vi "GRIPPER.vi"() -> ()   [LabVIEW 2016]
uses:
  <vilib>/myRIO/Instrument Drivers/Onboard IO/DIO/typedefs/DIO Reference.ctl
  <vilib>/myRIO/Common/Instrument Driver Framework/Utilities/typedefs/myRIO Generic Hardware Reference.ctl
  <vilib>/myRIO/Common/Instrument Driver Framework/Utilities/typedefs/Hardware Version Enum.ctl
  <vilib>/myRIO/Common/Instrument Driver Framework/Utilities/typedefs/myRIO v1.0 Reference.ctl
  <vilib>/myRIO/Common/Instrument Driver Framework/Utilities/typedefs/Generic FPGA Reference.ctl
  <vilib>/myRIO/Common/Instrument Driver Framework/myRIO v1.0/DIO/typedefs/DIO Channels List.ctl
  <vilib>/myRIO/Common/Instrument Driver Framework/myRIO v1.0/DIO/typedefs/DIO Channels Enum.ctl
  <vilib>/userdefined/High Color/nirio_resource_hc.ctl
  <vilib>/myRIO/Instrument Drivers/Onboard IO/AI/typedefs/AI Reference.ctl
  <vilib>/myRIO/Common/Instrument Driver Framework/myRIO v1.0/AI/typedefs/AI Channels List.ctl
  <vilib>/myRIO/Common/Instrument Driver Framework/myRIO v1.0/AI/typedefs/AI Channels Enum.ctl
  <vilib>/myRIO/Common/Instrument Driver Framework/Utilities/typedefs/Analog Scaling Constants List.ctl
  <vilib>/myRIO/Common/Instrument Driver Framework/Utilities/typedefs/Analog Scaling Constants.ctl
  <vilib>/myRIO/Common/Instrument Driver Framework/Utilities/vis/Is FPGA Ref Available.vi
  <vilib>/myRIO/Common/Instrument Driver Framework/myRIO v1.0/AI/vis/myRIO v1.1 Open AI.vi
  <vilib>/myRIO/Instrument Drivers/Onboard IO/AI/vis/Read.vi
  <vilib>/myRIO/Common/Instrument Driver Framework/myRIO v1.0/DIO/vis/myRIO v1.1 Open DIO.vi
  <vilib>/myRIO/Instrument Drivers/Onboard IO/DIO/vis/Write.vi
  <vilib>/myRIO/Common/Instrument Driver Framework/Utilities/vis/Validate Channels.vi
  <vilib>/myRIO/Common/Instrument Driver Framework/myRIO v1.0/AI/vis/myRIO v1.0 Reserve AI.vi
  <vilib>/myRIO/Common/Instrument Driver Framework/myRIO v1.0/DIO/vis/myRIO v1.0 Reserve DIO.vi
  <vilib>/myRIO/Common/Instrument Driver Framework/myRIO v1.0/PWM/vis/myRIO v1.1 Open PWM.vi
  <vilib>/myRIO/Common/Instrument Driver Framework/myRIO v1.0/UART/vis/myRIO v1.0 Close UART.vi
  <vilib>/myRIO/Common/Instrument Driver Framework/myRIO v1.0/AI/vis/myRIO v1.0 Build MUX Configuration AI.vi
  <vilib>/myRIO/Common/Instrument Driver Framework/myRIO v1.0/Resource Manager/vis/myRIO v1.0 Reserve Channel List.vi
  <vilib>/myRIO/Common/Instrument Driver Framework/myRIO v1.0/DIO/vis/myRIO v1.0 Build MUX Configuration DIO.vi
  <vilib>/myRIO/Common/Instrument Driver Framework/myRIO v1.0/PWM/vis/myRIO v1.0 Reserve PWM.vi
  <vilib>/myRIO/Common/Instrument Driver Framework/myRIO v1.0/Resource Manager/vis/myRIO v1.0 Reserve Channel.vi
  <vilib>/myRIO/Common/Instrument Driver Framework/myRIO v1.0/Resource Manager/vis/myRIO v1.0 Unreserve Channel.vi
  <vilib>/myRIO/Common/Instrument Driver Framework/myRIO v1.0/Resource Manager/vis/myRIO v1.0 Create Configuration List.vi
  <vilib>/myRIO/Common/Instrument Driver Framework/myRIO v1.0/PWM/vis/myRIO v1.0 Build MUX Configuration PWM.vi
  <vilib>/myRIO/Common/Instrument Driver Framework/myRIO v1.0/Resource Manager/vis/myRIO v1.0 Build Mutex Name.vi
  <vilib>/Utility/VariantDataType/GetNumericInfo.vi
  <vilib>/Utility/error.llb/Error Cluster From Error Code.vi
  <vilib>/myRIO/Common/Instrument Driver Framework/myRIO v1.0/myRIO v1.1 Open.vi
  <vilib>/myRIO/Common/Instrument Driver Framework/Utilities/vis/IO Manager.vi
  <vilib>/myRIO/Common/Instrument Driver Framework/Utilities/vis/Configuration Manager.vi
  <vilib>/myRIO/Common/Instrument Driver Framework/myRIO v1.0/Resource Manager/vis/myRIO v1.0 Configure IO.vi
  <vilib>/myRIO/Common/Instrument Driver Framework/myRIO v1.0/myRIO v1.0 Close.vi
  <vilib>/myRIO/Common/Instrument Driver Framework/myRIO v1.0/DIO/vis/myRIO v1.0 Write DIO.vi
  <vilib>/myRIO/Common/Instrument Driver Framework/myRIO v1.0/PWM/vis/myRIO v1.0 Write PWM.vi
  <vilib>/myRIO/Common/Instrument Driver Framework/myRIO v1.0/AI/vis/myRIO v1.0 Get Scaling Constants AI.vi
  <vilib>/myRIO/Common/Instrument Driver Framework/myRIO v1.0/AI/vis/myRIO v1.0 Read AI.vi
  <vilib>/myRIO/Common/Instrument Driver Framework/Utilities/vis/FPGA Ref Manager.vi
  <vilib>/myRIO/Common/Instrument Driver Framework/myRIO v1.0/myRIO v1.0 Reset FPGA.vi
  <vilib>/myRIO/Common/Instrument Driver Framework/myRIO v1.0/IRQ/vis/myRIO v1.0 IRQ Info FGV.vi
  <vilib>/myRIO/Common/Instrument Driver Framework/myRIO v1.0/IRQ/vis/myRIO v1.0 Timer IRQ Info FGV.vi
  <vilib>/myRIO/Common/Instrument Driver Framework/myRIO v1.0/IRQ/vis/myRIO v1.0 ISR Agent.vi
  <vilib>/myRIO/Express VI/Onboard IO/DO/DO Express VI.xnode
  <vilib>/myRIO/Instrument Drivers/Onboard IO/DIO/vis/myRIO DIO Open.xnode
  <vilib>/myRIO/Express VI/Onboard IO/AI/AI Express VI.xnode
  <vilib>/myRIO/Instrument Drivers/Onboard IO/AI/vis/myRIO AI Open.xnode
  <vilib>/myRIO/Instrument Drivers/Onboard IO/DIO/DIO.lvlib
  <vilib>/myRIO/Instrument Drivers/Onboard IO/AI/AI.lvlib
  <vilib>/myRIO/Instrument Drivers/Onboard IO/PWM/PWM.lvlib
  <vilib>/myRIO/Instrument Drivers/Utilities/Utilities.lvlib
panel:
  out "FSR 2":bool
  in  "Boolean":bool
  in  "milliseconds to wait 5":u32
  out "left fsr (A/AI1 (Pin 5))":dbl
  in  "Servo":bool
  in  "PWM channel":tag="B/PWM0"
  out "position [%FS]":dbl(slide) scale=0.0..180.0 scale format="%#_5g"
  out "pulse width [ms]":dbl=1.5
  out "duty cycle [%]":dbl
  in  "Stop Button":bool
  out "B/AI0 (Pin 3)":dbl
  out "Knob":dbl(knob) scale=0.0..4.0
  out "C Count":dbl
  out "A":bool
  out "C 2":bool
  out "D":bool
  out "B":bool
  in  "DIRECTION":bool
  in  "DRIVE":bool
  out "CC Count":dbl
  # "WHEN  THE DIRECTION BUTTON IS PRESSED \nTHE ROTATION IS COUNTER-CLOCK WISE"
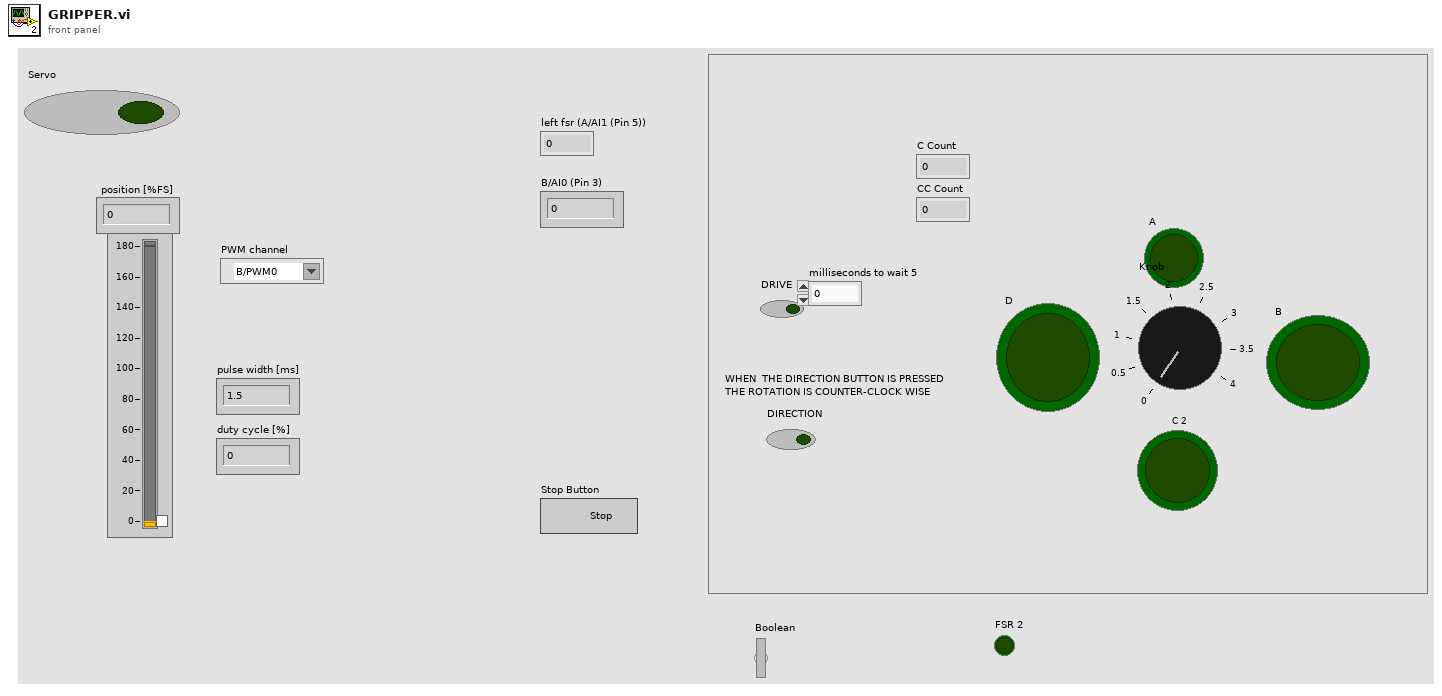
[diagram p1: front panel]
types:
  T1 = typedef "DIO.lvlib/DIO Reference.ctl" = cluster{"myRIO Reference":T2, "DIO Channels List":T6}
  T2 = typedef "myRIO Generic Hardware Reference.ctl" = cluster{"myRIO Model":T3, "myRIO Hardware Reference":T4}
  T3 = typedef "Hardware Version Enum.ctl" = enum16{"Unknown", "myRIO-1900", "myRIO-1950", "roboRIO", "NI ELVIS RIO CM"}
  T4 = typedef "myRIO v1.0 Reference.ctl" = cluster{"Generic FPGA Reference":T5, "Allow multiple opens":bool}
  T5 = typedef "Generic FPGA Reference.ctl" = refnum<k20>
  T6 = typedef "DIO Channels List.ctl" = T7[]
  T7 = typedef "DIO Channels Enum.ctl" = enum16{"Not Connected", "C/DIO0", "C/DIO1", "C/DIO2", "C/DIO3", "C/DIO4", "C/DIO5", "C/DIO6", "C/DIO7", "A/DIO0", "A/DIO1", "A/DIO2", "A/DIO3", "A/DIO4", "A/DIO5", "A/DIO6", "A/DIO7", "A/DIO8", "A/DIO9", "A/DIO10", "A/DIO11", "A/DIO12", "A/DIO13", "A/DIO14", "A/DIO15", "B/DIO0", "B/DIO1", "B/DIO2", "B/DIO3", "B/DIO4", "B/DIO5", "B/DIO6", "B/DIO7", "B/DIO8", "B/DIO9", "B/DIO10", "B/DIO11", "B/DIO12", "B/DIO13", "B/DIO14", "B/DIO15", "LED0", "LED1", "LED2", "LED3", "Button0", "DIO/DIO0", "DIO/DIO1", "DIO/DIO2", "DIO/DIO3", "DIO/DIO4", "DIO/DIO5", "DIO/DIO6", "DIO/DIO7", "DIO/DIO8", "DIO/DIO9", "SPI/CS0", "SPI/CS1", "SPI/CS2", "SPI/CS3", "LED RADIO (Green)", "LED RADIO (Red)", "LED COMM (Green)", "LED COMM (Red)", "LED MODE (Green)", "LED MODE (Red)"}
  T8 = typedef "nirio_resource_hc.ctl" = tag
  T9 = typedef "AI.lvlib/AI Reference.ctl" = cluster{"myRIO Reference":T2, "AI Channels List":T10, "AI Scaling Constants List":T12}
  T10 = typedef "AI Channels List.ctl" = T11[]
  T11 = typedef "AI Channels Enum.ctl" = enum16{"Not Connected", "AudioIn/Left", "AudioIn/Right", "C/AI0", "C/AI1", "A/AI0", "A/AI1", "A/AI2", "A/AI3", "B/AI0", "B/AI1", "B/AI2", "B/AI3", "AI/AI0", "AI/AI1", "AI/AI2", "AI/AI3"}
  T12 = typedef "Analog Scaling Constants List.ctl" = T13[]
  T13 = typedef "Analog Scaling Constants.ctl" = cluster{"LSB Weight (Volts)":dbl, "Offset (Volts)":dbl, "Signed?":bool}
  T14 = typedef "PWM.lvlib/PWM Reference.ctl" = cluster{"myRIO Reference":T2, "PWM Channels Enum":T15, "PWM Configuration":T16}
  T15 = typedef "PWM Channels Enum.ctl" = enum16{"Not Connected", "C/PWM0", "C/PWM1", "A/PWM0", "A/PWM1", "A/PWM2", "B/PWM0", "B/PWM1", "B/PWM2", "PWM/PWM0", "PWM/PWM1", "PWM/PWM2", "PWM/PWM3", "PWM/PWM4", "PWM/PWM5", "PWM/PWM6", "PWM/PWM7", "PWM/PWM8", "PWM/PWM9"}
  T16 = typedef "PWM.lvlib/PWM Configuration.ctl" = cluster{"Frequency":dbl, "Duty Cycle":dbl}
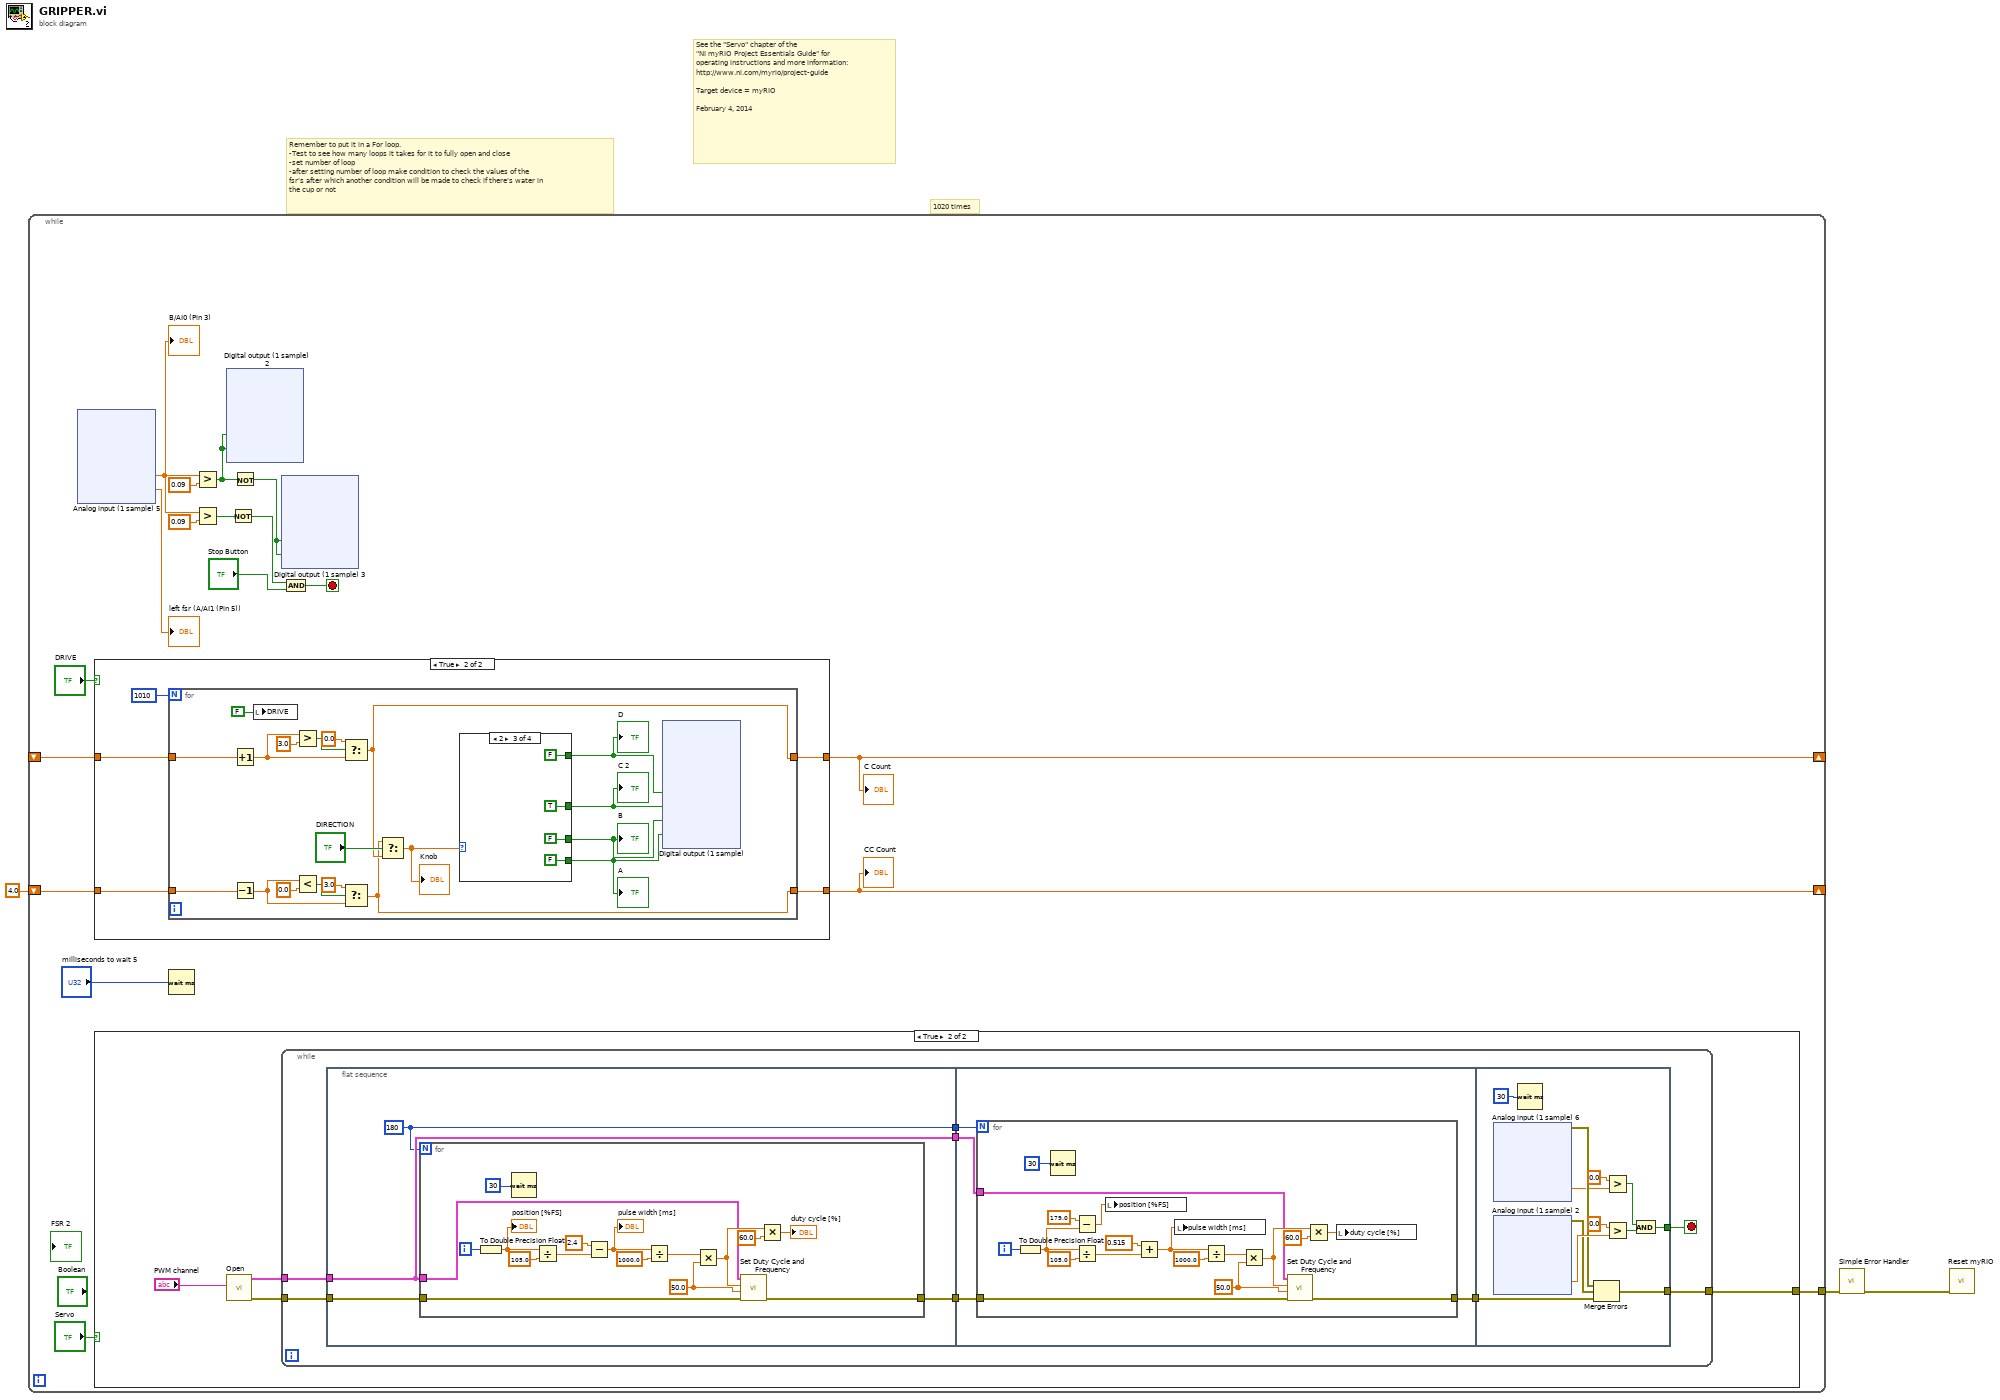
[diagram p0: block diagram]
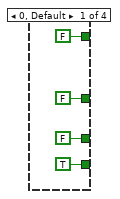
[diagram p3: hidden frame]
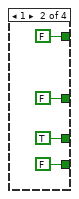
[diagram p4: hidden frame]
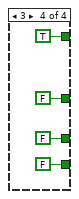
[diagram p5: hidden frame]
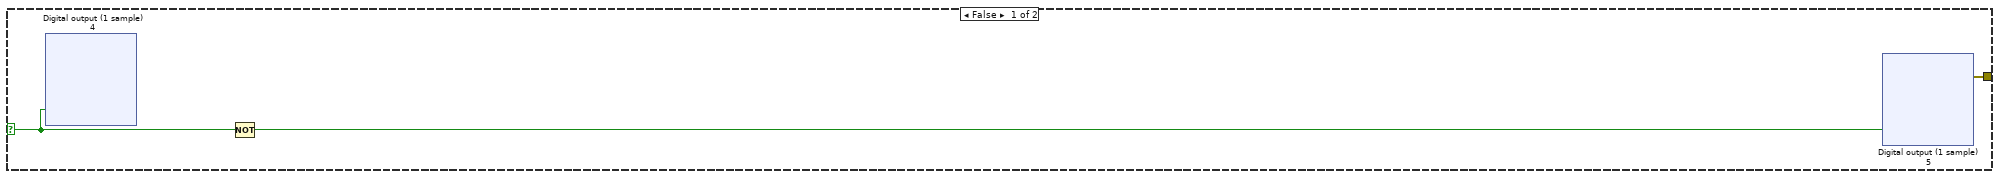
[diagram p6: hidden frame]
diagram:
  # "1020 times"
  # "Remember to put it in a For loop.\n-Test to see how many loops it takes for it to fully open and close\n-set number of loop\n-after setting number of loop make condition to check the values of the \nfsr's after which another condition will be made to check if there's water in \nthe cup or not"
  # "See the \"Servo\" chapter of the\n\"NI myRIO Project Essentials Guide\" for\noperating instructions and more information: \nhttp://www.ni.com/myrio/project-guide\n\nTarget device = myRIO\n\nFebruary 4, 2014"
  n1 = while {
    tunnel: [w21] -> w2
    shift-right: [w7] -> _
    shift-left: 4.0 -> [w20]
    shift-right: [w4] -> _
    shift-left: _ -> [w19]
    stop <- w13 stop-if-true
    n2 = xnode "Analog input (1 sample) 5"() -> ("right fsr (A/AI0 (Pin 3))"=w9:dbl, "left fsr (A/AI1 (Pin 5))"=→"left fsr (A/AI1 (Pin 5))":dbl)  [unwired: 1 in, 1 out]
    "B/AI0 (Pin 3)" <- w9
    n3 = case shown="True" "DRIVE" {
      tunnel: w20 -> [w23 w28]
      tunnel: w19 -> [w22 w27]
      tunnel: [w22 w26] -> w4
      tunnel: [w23 w25] -> w7
      frame False {
      }
      frame True {
        n4 = for {
          N: 1010 -> [_]
          tunnel: w28 -> [w33]
          tunnel: w27 -> [w32]
          tunnel: [w31] -> w26
          tunnel: [w30] -> w25
          n5 = Increment(x=w32) -> (x+1=w39:dbl)
          n6 = Decrement(x=w33) -> (x-1=w40:dbl)
          n7 = local write "DRIVE"(FALSE) -> ()
          n8 = Greater?(x=w39, y=3.0) -> (0:w43:bool)
          n9 = Less?(x=w40, y=0.0) -> (x < y?=w46:bool)
          n10 = Select(t=0.0, s=w43, f=w39) -> (s? t:f=w31:dbl)
          n11 = Select(t=3.0, s=w46, f=w40) -> (s? t:f=w30:dbl)
          n12 = Select(t=w30, s="DIRECTION", f=w31) -> (s? t:f=w34:dbl)
          "Knob" <- w34
          n13 = case shown="2" w34 {
            tunnel: [TRUE FALSE FALSE FALSE] -> w38
            tunnel: [FALSE FALSE FALSE TRUE] -> w35
            tunnel: [FALSE FALSE TRUE FALSE] -> w36
            tunnel: [FALSE TRUE FALSE FALSE] -> w37
            frame 0, Default {
            }
            frame 1 {
            }
            frame 2 {
            }
            frame 3 {
            }
          }
          "A" <- w38
          "C 2" <- w36
          "D" <- w35
          "B" <- w37
          n14 = xnode "Digital output (1 sample)"("IN4 (A/DIO10 (Pin 31))"=w35, "IN3 (A/DIO11 (Pin 18))"=w36, "IN2 (A/DIO13 (Pin 26))"=w37, "IN1 (A/DIO15 (Pin 34))"=w38) -> ()  [unwired: 1 in, 1 out]
        }
      }
    }
    "C Count" <- w4
    "CC Count" <- w7
    n15 = case shown="True" "Servo" {
      selector: "Servo" -> [w212 _]
      tunnel: [w213 w286] -> w21
      frame False {
        n16 = xnode "Digital output (1 sample) 4"("B/DIO15 (Pin 34)"=w212) -> ()  [unwired: 1 in, 1 out]
        n17 = Not(x=w212) -> (.not. x?=w214:bool)
        n18 = xnode "Digital output (1 sample) 5"("B/DIO14 (Pin 32)"=w214) -> ("error out"=w213:errorcluster)  [unwired: 1 in]
      }
      frame True {
        n19 = call <vilib>:"Open.vi"("Channel Name"="PWM channel") -> ("error out"=w285:errorcluster, "PWM Ref Out"=w287:T14)  [unwired: 9 in]
        n20 = while {
          tunnel: w287 -> [w296]
          tunnel: [w291] -> w286
          tunnel: w285 -> [w295]
          stop <- w289 stop-if-true
          n21 = flat-sequence {
            tunnel: w296 -> [w298]
            tunnel: w295 -> [w299]
            tunnel: [w300] -> w294
            tunnel: [w298] -> w293
            tunnel: [w297] -> w292
            tunnel: w294 -> [w318]
            tunnel: w293 -> [w320]
            tunnel: w292 -> [w319]
            tunnel: [w317] -> w290
            tunnel: [w344] -> w291
            tunnel: w290 -> [w345]
            tunnel: [w348] -> w289
            frame #0 {
              w297 = 180
              n22 = for {
                N: w297 -> [_]
                tunnel: [w312] -> w300
                tunnel: w298 -> [w304]
                tunnel: w299 -> [w301]
                i -> [w302]
                w313 = 50.0 ("freq [Hz]")
                n23 = To Double Precision Float(number=w302) -> (double precision float=w305:dbl)
                "position [%FS]" <- w305
                n24 = Wait (ms)(milliseconds to wait=u32 30) -> ()  [unwired: 1 out]
                n25 = Divide(x=w305, y=105.0) -> (x/y=w307:dbl)
                n26 = Subtract(x=2.4 ("y"), y=w307) -> (x-y=w303:dbl)
                "pulse width [ms]" <- w303
                n27 = Divide(x=w303, y=1000.0) -> (x/y=w311:dbl)
                n28 = Multiply(x=w311, y=w313) -> (x*y=w308:dbl)
                n29 = call <vilib>:"Set Duty Cycle and Frequency.vi"("error in (no error)"=w301, "Frequency [Hz]"=w313, "Duty Cycle"=w308, "PWM Ref In"=w304) -> ("error out"=w312:errorcluster)  [unwired: 5 in, 1 out]
                n30 = Multiply(x=w308, y=60.0) -> (x*y=→"duty cycle [%]":dbl)
              }
            }
            frame #1 {
              n31 = for {
                N: w319 -> [_]
                tunnel: [w334] -> w317
                tunnel: w318 -> [w327]
                tunnel: w320 -> [w326]
                i -> [w328]
                w335 = 50.0 ("freq [Hz]")
                n32 = To Double Precision Float(number=w328) -> (double precision float=w322:dbl)
                n33 = Wait (ms)(milliseconds to wait=u32 30) -> ()  [unwired: 1 out]
                n34 = Subtract(x=179.0, y=w322) -> (x-y=w323:dbl)
                n35 = Divide(x=w322, y=105.0) -> (x/y=w330:dbl)
                n36 = local write "position [%FS]"(w323) -> ()
                n37 = Add(x=0.515 ("y"), y=w330) -> (x+y=w325:dbl)
                n38 = local write "pulse width [ms]"(w325) -> ()
                n39 = Divide(x=w325, y=1000.0) -> (x/y=w333:dbl)
                n40 = Multiply(x=w333, y=w335) -> (x*y=w331:dbl)
                n41 = call <vilib>:"Set Duty Cycle and Frequency.vi"("error in (no error)"=w327, "Frequency [Hz]"=w335, "Duty Cycle"=w331, "PWM Ref In"=w326) -> ("error out"=w334:errorcluster)  [unwired: 5 in, 1 out]
                n42 = Multiply(x=w331, y=60.0) -> (x*y=w324:dbl)
                n43 = local write "duty cycle [%]"(w324) -> ()
              }
            }
            frame #2 {
              n44 = xnode "Analog input (1 sample) 6"() -> ("B/AI0 (Pin 3)"=w343:dbl, "error out"=w347:errorcluster)  [unwired: 1 in]
              n45 = xnode "Analog input (1 sample) 2"() -> ("A/AI1 (Pin 5)"=w349:dbl, "error out"=w346:errorcluster)  [unwired: 1 in]
              n46 = Wait (ms)(milliseconds to wait=u32 30) -> ()  [unwired: 1 out]
              n47 = Merge Errors(w347, w346, w345) -> (w344:errorcluster)
              n48 = Greater?(x=0.0, y=w343) -> (0:w342:bool)
              n49 = Greater?(x=0.0, y=w349) -> (0:w350:bool)
              n50 = And(x=w342, y=w350) -> (x .and. y?=w348:bool)
            }
          }
        }
      }
    }
    n51 = Wait (ms)(milliseconds to wait="milliseconds to wait 5") -> ()  [unwired: 1 out]
    n52 = Greater?(x=w9, y=0.09) -> (0:w14:bool)
    n53 = Greater?(x=w9, y=0.09) -> (0:w8:bool)
    n54 = xnode "Digital output (1 sample) 2"("GREEN-LED (A/DIO0 (Pin 11))"=w14, "GREEN-LED1 (A/DIO1 (Pin 13))"=w14) -> ()  [unwired: 1 in, 1 out]
    n55 = Not(x=w8) -> (.not. x?=w12:bool)
    n56 = Not(x=w14) -> (.not. x?=w17:bool)
    n57 = xnode "Digital output (1 sample) 3"("RED-LED1 (A/DIO5 (Pin 21))"=w17, "RED-LED2 (A/DIO6 (Pin 23))"=w17) -> ()  [unwired: 1 in, 1 out]
    n58 = And(x=w12, y="Stop Button") -> (x .and. y?=w13:bool)
  }
  n59 = call <vilib>:"Simple Error Handler.vi"("error in (no error)"=w2) -> ("error out"=w3:errorcluster)  [unwired: 4 in, 4 out]
  n60 = call <vilib>:"Reset myRIO.vi"("error in (no error)"=w3) -> ()  [unwired: 10 in, 1 out]
